vi "UTIL_Get Queue Token String v1_0_0.vi"(7 "timeout in ms (-1)":i32=-1, 8 "error in (no error)":errorcluster, 9 "Token":string[](array[string])=["?"], 11 "queue":refnum<queue>) -> (0 "error out":errorcluster, 1 "token string":string, 2 "timed out?":bool, 3 "queue out":refnum<queue>, 4 "dup string":string, 5 "dup - token string":string, 6 "offset past token":i32)   [LabVIEW 2015]
doc: "UTIL_Get Queue Token String v1_0_0.vi\n\nNormal dequeue element vi with the addition of scan string for tokens. Allows use for a 3D state machine.\n\nCreated 2006 by\nJ. Daren Suntych\nNational Analytics\n970-397-0764"
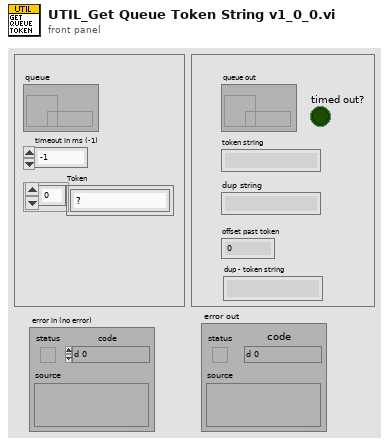
[diagram p1: front panel]
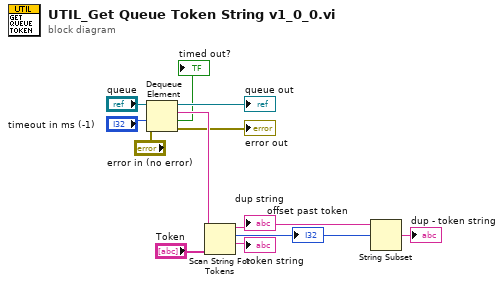
[diagram p0: block diagram]
diagram:
  n1 = Dequeue Element(queue="queue", timeout in ms (-1)="timeout in ms (-1)", error in (no error)="error in (no error)") -> (queue out=→"queue out":refnum<queue>, element=w12:string, timed out?=→"timed out?":bool, error out=→"error out":errorcluster)
  n2 = Scan String For Tokens(6:"Token", 9:w12) -> (1:→"token string":string, 2:w1:i32, 3:w2:string)  [unwired: 1 in, 4 out]
  "dup string" <- w2
  "offset past token" <- w1
  n3 = String Subset(string=w2, offset (0)=w1) -> (substring=→"dup - token string":string)  [unwired: 1 out]
